vi "HDF5_Init_UPS_Refs.vi"(5 "HDF5 file ref":T3 format="%.0x", 9 "File Exists?":bool, 11 "error in":errorcluster) -> (4 "UPS_refs":T1 {"TimeStamp_dset" format="%.0x"; "TimeString_dset" format="%.0x"; "%_dset" format="%.0x"; "W_dset" format="%.0x"; "Hz_dset" format="%.0x"; "A_dset" format="%.0x"; "V_dset" format="%.0x"; "Group_ref" format="%.0x"}, 6 "HDF5 file ref":T3 format="%.0x", 15 "error out":errorcluster)   [LabVIEW 2018]
doc: "Set up the HDF5 data structure and initialize the references for the Tone1, Tone2, Tone3, and Tone4 Groups and the datasets (tables) within each Group.\n\nData structure:\nTone1 (Group) \n Beac - cluster (Dataset)\n BeacZoom - 1024 element Double array (waveform) \n Cal - cluster\n CalZoom - 1024 element Double array (waveform) \nTone2\n Beac - cluster\n BeacZoom - 1024 element Double array (waveform) \n Cal - cluster\n CalZoom - 1024 element Double array (waveform) \nTone3\n Beac - cluster\n BeacZoom - 1024 element Double array (waveform) \n Cal - cluster\n CalZoom - 1024 element Double array (waveform) \nTone4\n Beac - cluster\n BeacZoom - 1024 element Double array (waveform) \n Cal - cluster\n CalZoom - 1024 element Double array (waveform)"
uses:
  <vilib>/addons/h5labview2/group/H5G.lvlib
  <vilib>/addons/h5labview2/dataset/H5D.lvlib
  <vilib>/addons/h5labview2/base/hid_t_renamed.ctl
  UPS_refs.ctl
  <vilib>/addons/h5labview2/base/hid_t.ctl
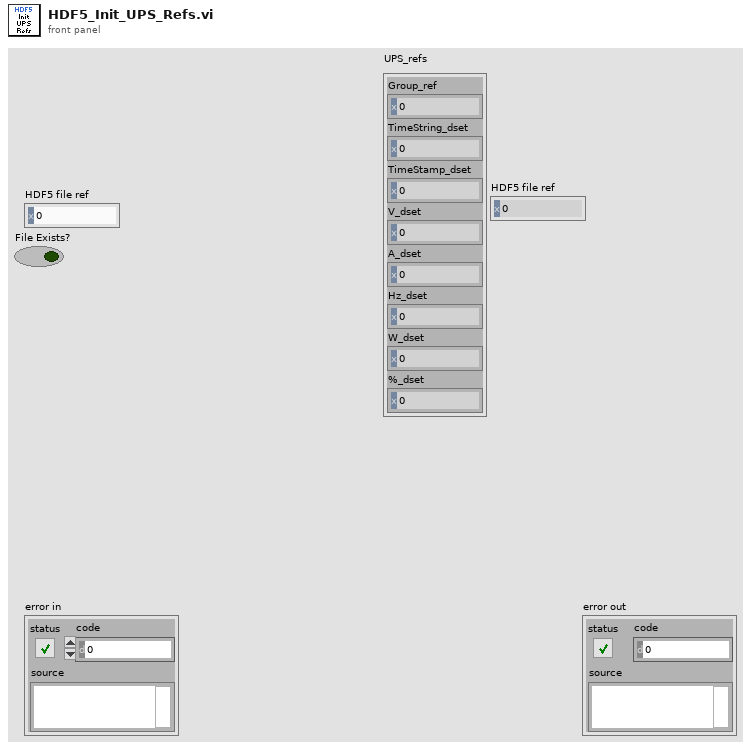
[diagram p1: front panel]
types:
  T1 = typedef "UPS_refs.ctl" = cluster{"Group_ref":T2, "TimeString_dset":T2, "TimeStamp_dset":T2, "V_dset":T2, "A_dset":T2, "Hz_dset":T2, "W_dset":T2, "%_dset":T2}
  T2 = typedef "hid_t.ctl" = i32
  T3 = typedef "hid_t_renamed.ctl" = i32
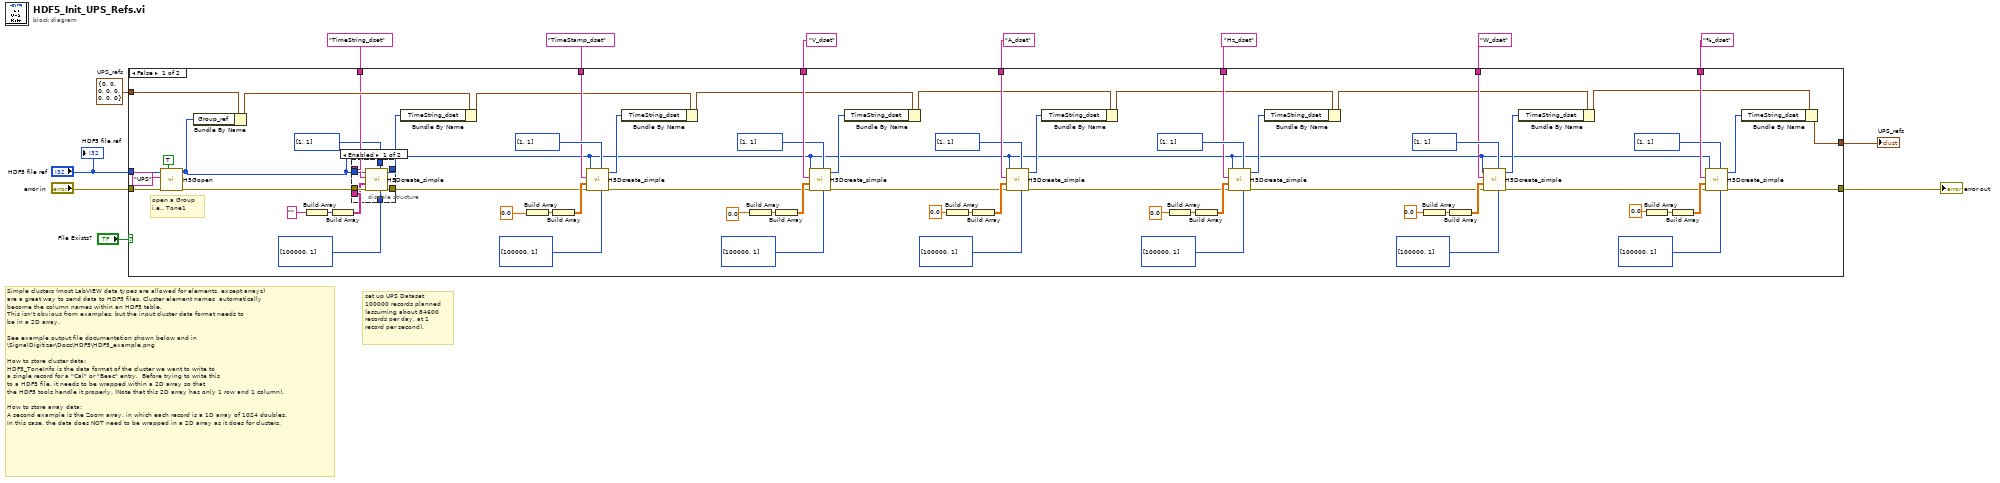
[diagram p0: block diagram]
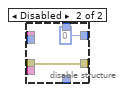
[diagram p2: hidden frame]
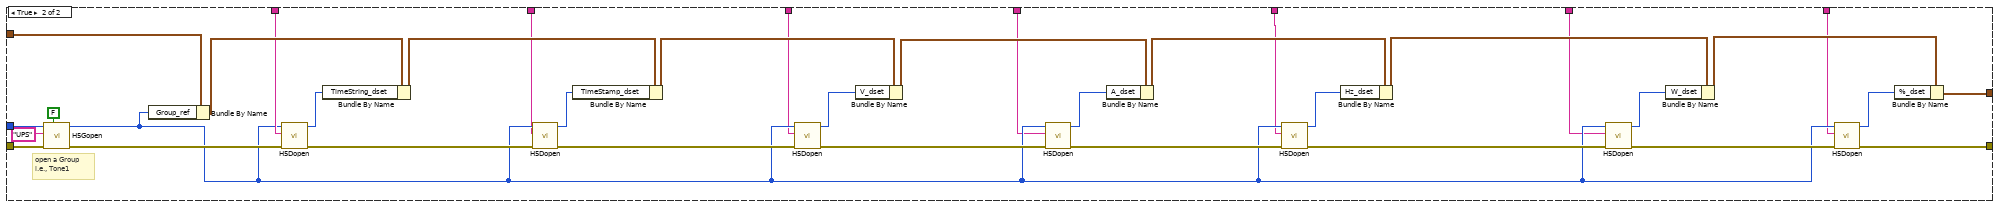
[diagram p3: hidden frame]
diagram:
  w9 = T1 {"Group_ref"=0, "TimeString_dset"=0, "TimeStamp_dset"=0, "V_dset"=0, "A_dset"=0, "Hz_dset"=0, "W_dset"=0, "%_dset"=0}  # UPS_refs
  # "set up UPS Dataset\n100000 records planned\n(assuming about 84600\nrecords per day, at 1\nrecord per second)."
  # "Simple clusters (most LabVIEW data types are allowed for elements, except arrays) \nare a great way to send data to HDF5 files. Cluster element names  automatically\nbecome the column names within an HDF5 table.\nThis isn't obvious from examples, but the input cluster data format needs to \nbe in a 2D array.\n\nSee example output file documentation shown below and in\n\\SignalDigitizer\\Docs\\HDF5\\HDF5_example.png\n\nHow to store cluster data:\nHDF5_ToneInfo is the data format of the cluster we want to write to \na single record for a \"Cal\" or \"Beac\" entry.  Before trying to write this \nto a HDF5 file, it needs to be wrapped within a 2D array so that \nthe HDF5 tools handle it properly. (Note that this 2D array has only 1 row and 1 column).\n\nHow to store array data:\nA second example is the Zoom array, in which each record is a 1D array of 1024 doubles.\nIn this case, the data does NOT need to be wrapped in a 2D array as it does for clusters."
  n1 = case shown="False" "File Exists?" {
    tunnel: "error in" -> [w84 w130]
    tunnel: "HDF5 file ref" -> [w83 w129]
    tunnel: [w34 w109] -> w11
    tunnel: w9 -> [w78 w124]
    tunnel: [w20 w102] -> w8
    tunnel: "TimeString_dset" ("string") -> [w73 w122]
    tunnel: "TimeStamp_dset" ("string") -> [w65 w95]
    tunnel: "V_dset" ("string") -> [w64 w96]
    tunnel: "A_dset" ("string") -> [w52 w100]
    tunnel: "Hz_dset" ("string") -> [w53 w99]
    tunnel: "W_dset" ("string") -> [w41 w98]
    tunnel: "%_dset" ("string") -> [w40 w97]
    frame False {
      # "open a Group\ni.e., Tone1"
      n2 = call <vilib>:"H5Gopen.vi"("create? (F)"=TRUE, "error in (no error)"=w84, "name"="UPS", "ref in"=w83) -> ("error out"=w81:errorcluster, "group out"=w27:T2)  [unwired: 6 in]
      n3 = Bundle By Name(cluster=w78, "Group_ref"=w27) -> (w80:T1)
      n4 = Build Array("" ("TimeString")) -> (w76:string[])
      n5 = Build Array(w76) -> (w75:string[][])
      n6 = disable-structure shown="Enabled" {
        disable-tunnel: w81 -> [w92 w94]
        disable-tunnel: [w91 T3 0 ("dset out")] -> w79
        disable-tunnel: w75 -> [w90 _]
        disable-tunnel: u64[] [100000, 1] ("max size") -> [w89 _]
        disable-tunnel: w73 -> [w88 _]
        disable-tunnel: i32[] [1, 1] ("size(s)") -> [w87 _]
        disable-tunnel: [w86 w94] -> w28
        disable-tunnel: w27 -> [w85 _]
        frame Enabled {
          n7 = call <vilib>:"H5Dcreate_simple.vi"("max size"=w89, "chunk size"=w87, "error in (no error)"=w92, "type in"=w90, "name"=w88, "ref in"=w85) -> ("error out"=w86:errorcluster, "dset out"=w91:T2)  [unwired: 4 in]
        }
        frame Disabled {
        }
      }
      n8 = Bundle By Name(cluster=w80, "TimeString_dset"=w79) -> (w26:T1)
      n9 = Build Array(0.0 ("TimeStamp")) -> (w67:dbl[])
      n10 = Build Array(w67) -> (w68:dbl[][])
      n11 = call <vilib>:"H5Dcreate_simple.vi"("max size"=u64[] [100000, 1], "chunk size"=i32[] [1, 1] ("size(s)"), "error in (no error)"=w28, "type in"=w68, "name"=w65, "ref in"=w27) -> ("error out"=w29:errorcluster, "dset out"=w66:T2)  [unwired: 4 in]
      n12 = Bundle By Name(cluster=w26, "TimeString_dset"=w66) -> (w25:T1)
      n13 = Build Array(0.0 ("V")) -> (w62:dbl[])
      n14 = Build Array(w62) -> (w61:dbl[][])
      n15 = call <vilib>:"H5Dcreate_simple.vi"("max size"=u64[] [100000, 1], "chunk size"=i32[] [1, 1] ("size(s)"), "error in (no error)"=w29, "type in"=w61, "name"=w64, "ref in"=w27) -> ("error out"=w30:errorcluster, "dset out"=w63:T2)  [unwired: 4 in]
      n16 = Bundle By Name(cluster=w25, "TimeString_dset"=w63) -> (w24:T1)
      n17 = Build Array(0.0 ("A")) -> (w50:dbl[])
      n18 = Build Array(w50) -> (w49:dbl[][])
      n19 = call <vilib>:"H5Dcreate_simple.vi"("max size"=u64[] [100000, 1], "chunk size"=i32[] [1, 1] ("size(s)"), "error in (no error)"=w30, "type in"=w49, "name"=w52, "ref in"=w27) -> ("error out"=w31:errorcluster, "dset out"=w51:T2)  [unwired: 4 in]
      n20 = Bundle By Name(cluster=w24, "TimeString_dset"=w51) -> (w23:T1)
      n21 = Build Array(0.0 ("Hz")) -> (w55:dbl[])
      n22 = Build Array(w55) -> (w56:dbl[][])
      n23 = call <vilib>:"H5Dcreate_simple.vi"("max size"=u64[] [100000, 1], "chunk size"=i32[] [1, 1] ("size(s)"), "error in (no error)"=w31, "type in"=w56, "name"=w53, "ref in"=w27) -> ("error out"=w32:errorcluster, "dset out"=w54:T2)  [unwired: 4 in]
      n24 = Bundle By Name(cluster=w23, "TimeString_dset"=w54) -> (w22:T1)
      n25 = Build Array(0.0 ("W")) -> (w43:dbl[])
      n26 = Build Array(w43) -> (w44:dbl[][])
      n27 = call <vilib>:"H5Dcreate_simple.vi"("max size"=u64[] [100000, 1], "chunk size"=i32[] [1, 1] ("size(s)"), "error in (no error)"=w32, "type in"=w44, "name"=w41, "ref in"=w27) -> ("error out"=w33:errorcluster, "dset out"=w42:T2)  [unwired: 4 in]
      n28 = Bundle By Name(cluster=w22, "TimeString_dset"=w42) -> (w21:T1)
      n29 = Build Array(0.0 ("%")) -> (w38:dbl[])
      n30 = Build Array(w38) -> (w37:dbl[][])
      n31 = call <vilib>:"H5Dcreate_simple.vi"("max size"=u64[] [100000, 1], "chunk size"=i32[] [1, 1] ("size(s)"), "error in (no error)"=w33, "type in"=w37, "name"=w40, "ref in"=w27) -> ("error out"=w34:errorcluster, "dset out"=w39:T2)  [unwired: 4 in]
      n32 = Bundle By Name(cluster=w21, "TimeString_dset"=w39) -> (w20:T1)
    }
    frame True {
      # "open a Group\ni.e., Tone1"
      n33 = call <vilib>:"H5Gopen.vi"("create? (F)"=FALSE, "error in (no error)"=w130, "name"="UPS", "ref in"=w129) -> ("error out"=w127:errorcluster, "group out"=w101:T2)  [unwired: 6 in]
      n34 = Bundle By Name(cluster=w124, "Group_ref"=w101) -> (w126:T1)
      n35 = call <vilib>:"H5Dopen.vi"("error in (no error)"=w127, "name"=w122, "loc in"=w101) -> ("error out"=w115:errorcluster, "dset out"=w125:T2)  [unwired: 7 in]
      n36 = Bundle By Name(cluster=w126, "TimeString_dset"=w125) -> (w108:T1)
      n37 = call <vilib>:"H5Dopen.vi"("error in (no error)"=w115, "name"=w95, "loc in"=w101) -> ("error out"=w114:errorcluster, "dset out"=w121:T2)  [unwired: 7 in]
      n38 = Bundle By Name(cluster=w108, "TimeStamp_dset"=w121) -> (w107:T1)
      n39 = call <vilib>:"H5Dopen.vi"("error in (no error)"=w114, "name"=w96, "loc in"=w101) -> ("error out"=w113:errorcluster, "dset out"=w119:T2)  [unwired: 7 in]
      n40 = Bundle By Name(cluster=w107, "V_dset"=w119) -> (w106:T1)
      n41 = call <vilib>:"H5Dopen.vi"("error in (no error)"=w113, "name"=w100, "loc in"=w101) -> ("error out"=w112:errorcluster, "dset out"=w120:T2)  [unwired: 7 in]
      n42 = Bundle By Name(cluster=w106, "A_dset"=w120) -> (w105:T1)
      n43 = call <vilib>:"H5Dopen.vi"("error in (no error)"=w112, "name"=w99, "loc in"=w101) -> ("error out"=w111:errorcluster, "dset out"=w118:T2)  [unwired: 7 in]
      n44 = Bundle By Name(cluster=w105, "Hz_dset"=w118) -> (w104:T1)
      n45 = call <vilib>:"H5Dopen.vi"("error in (no error)"=w111, "name"=w98, "loc in"=w101) -> ("error out"=w110:errorcluster, "dset out"=w117:T2)  [unwired: 7 in]
      n46 = Bundle By Name(cluster=w104, "W_dset"=w117) -> (w103:T1)
      n47 = call <vilib>:"H5Dopen.vi"("error in (no error)"=w110, "name"=w97, "loc in"=w101) -> ("error out"=w109:errorcluster, "dset out"=w116:T2)  [unwired: 7 in]
      n48 = Bundle By Name(cluster=w103, "%_dset"=w116) -> (w102:T1)
    }
  }
  "error out" <- w11
  "UPS_refs" <- w8
  "HDF5 file ref" <- "HDF5 file ref"
